vi "TextLimitToValueLimit.vi"(2 "min":string, 3 "max":string) -> (16 "min":dbl, 17 "max":dbl)   [LabVIEW 2018]
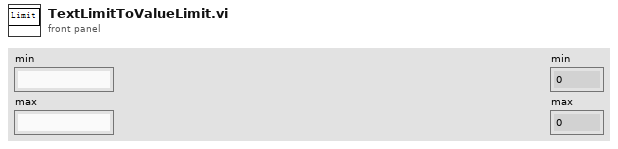
[diagram p1: front panel]
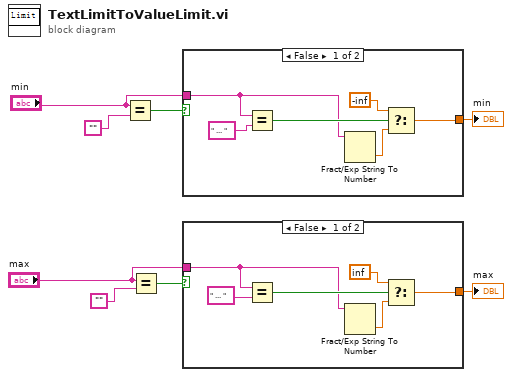
[diagram p0: block diagram]
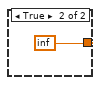
[diagram p2: hidden frame]
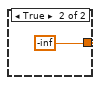
[diagram p3: hidden frame]
diagram:
  n1 = Equal?(x="min", y="") -> (x = y?=w6:bool)
  n2 = Equal?(x="max", y="") -> (x = y?=w3:bool)
  n3 = case shown="False" w6 {
    tunnel: "min" -> [w12 _]
    tunnel: [w11 -inf] -> w2
    frame False {
      n4 = Equal?(x=w12, y=" ... " ("f")) -> (x = y?=w13:bool)
      n5 = Fract/Exp String To Number(string=w12) -> (number=w10:dbl)  [unwired: 3 in, 1 out]
      n6 = Select(t=-inf, s=w13, f=w10) -> (s? t:f=w11:dbl)
    }
    frame True {
    }
  }
  "min" <- w2
  n7 = case shown="False" w3 {
    tunnel: "max" -> [w19 _]
    tunnel: [w18 inf] -> w1
    frame False {
      n8 = Equal?(x=w19, y=" ... " ("f")) -> (x = y?=w20:bool)
      n9 = Fract/Exp String To Number(string=w19) -> (number=w17:dbl)  [unwired: 3 in, 1 out]
      n10 = Select(t=inf, s=w20, f=w17) -> (s? t:f=w18:dbl)
    }
    frame True {
    }
  }
  "max" <- w1
